vi "Variant2Boolean.vi"(4 "Data":variant) -> (1 "Boolean":bool)   [LabVIEW 2016, in "System.lvlib"]
uses:
  System.lvlib
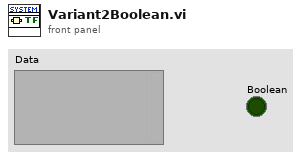
[diagram p1: front panel]
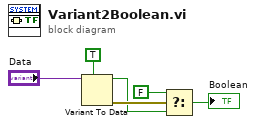
[diagram p0: block diagram]
diagram:
  n1 = Variant To Data(type=TRUE, Variant="Data") -> (data=w3:bool, error out=w4:errorcluster)  [unwired: 1 in]
  n2 = Select(t=FALSE, s=w4, f=w3) -> (s? t:f=→"Boolean":bool)
